vi "SpinCoaterArray2String_v03.vi"(3 "Time Start":dbl[unit], 4 "Program Spin Coater\nSpeed (rpm)          Time (s)":dbl[][](array[numeric])) -> (0 "Prg Spin Coater small":dbl[][](array[numeric]), 1 "remote control String":string)   [LabVIEW 2018, in "SpinCoater.lvclass"]
uses:
  <instrlib>/Classes/SpinCoater/SpinCoater.lvclass
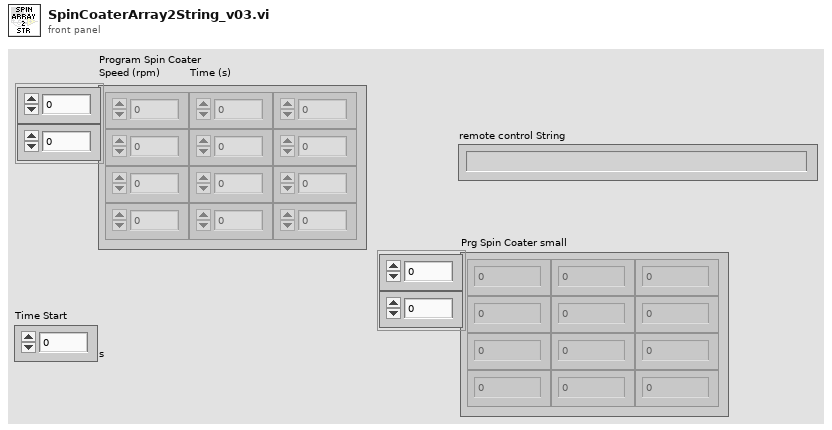
[diagram p1: front panel]
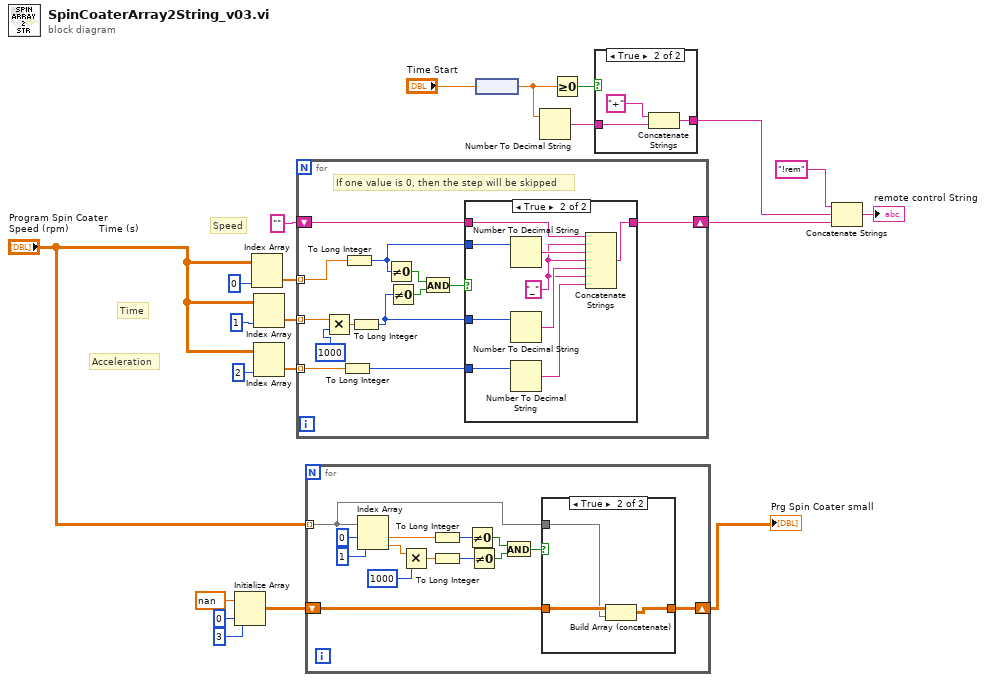
[diagram p0: block diagram]
diagram:
  # "Acceleration"
  # "Time"
  # "Speed"
  n1 = Initialize Array(nan ("element"), 0 ("dimension size"), 3 ("dimension size")) -> (w2:dbl[][])
  n2 = Index Array(array="Program Spin Coater\nSpeed (rpm)          Time (s)", index (col)=0 ("disabled index (col)")) -> (element=w19:dbl[])  [unwired: 1 in]
  n3 = Index Array(array="Program Spin Coater\nSpeed (rpm)          Time (s)", index (col)=1 ("disabled index (col)")) -> (element=w18:dbl[])  [unwired: 1 in]
  n4 = Index Array(array="Program Spin Coater\nSpeed (rpm)          Time (s)", index (col)=2 ("disabled index (col)")) -> (element=w7:dbl[])  [unwired: 1 in]
  n5 = for {
    tunnel: w19 -> [w31] mode=indexing
    tunnel: w18 -> [w24] mode=indexing
    shift-right: [w28] -> w9
    shift-left: "" ("string") -> [w29]
    tunnel: w7 -> [w27] mode=indexing
    # "If one value is 0, then the step will be skipped"
    n6 = Multiply(x=w24, y=1000) -> (x*y=w25:dbl)
    n7 = To Long Integer(number=w27) -> (32bit integer=w26:i32)
    n8 = To Long Integer(number=w31) -> (32bit integer=w30:i32)
    n9 = To Long Integer(number=w25) -> (32bit integer=w22:i32)
    n10 = Not Equal To 0?(x=w30) -> (x != 0?=w34:bool)
    n11 = Not Equal To 0?(x=w22) -> (x != 0?=w33:bool)
    n12 = And(x=w34, y=w33) -> (x .and. y?=w32:bool)
    n13 = case shown="True" w32 {
      tunnel: w30 -> [_ w44]
      tunnel: w22 -> [_ w43]
      tunnel: w29 -> [w35 w40]
      tunnel: [w35 w39] -> w28
      tunnel: w26 -> [_ w38]
      frame False {
      }
      frame True {
        w37 = "_" ("string")
        n14 = Number To Decimal String(number=w44) -> (decimal integer string=w42:string)  [unwired: 1 in]
        n15 = Number To Decimal String(number=w43) -> (decimal integer string=w41:string)  [unwired: 1 in]
        n16 = Number To Decimal String(number=w38) -> (decimal integer string=w36:string)  [unwired: 1 in]
        n17 = Concatenate Strings(w40, w37, w42, w37, w41, w37, w36) -> (w39:string)
      }
    }
  }
  n18 = for {
    tunnel: "Program Spin Coater\nSpeed (rpm)          Time (s)" -> [w50] mode=indexing
    shift-right: [w48] -> w1
    shift-left: w2 -> [w49]
    n19 = Index Array(array=w50, index #1=0 ("index"), index #2=1 ("index")) -> (element #1=w56:dbl, element #2=w46:dbl)
    n20 = Multiply(x=w46, y=1000) -> (x*y=w47:dbl)
    n21 = To Long Integer(number=w56) -> (32bit integer=w52:i32)
    n22 = To Long Integer(number=w47) -> (32bit integer=w53:i32)
    n23 = Not Equal To 0?(x=w52) -> (x != 0?=w55:bool)
    n24 = Not Equal To 0?(x=w53) -> (x != 0?=w54:bool)
    n25 = And(x=w55, y=w54) -> (x .and. y?=w51:bool)
    n26 = case shown="True" w51 {
      tunnel: w50 -> [_ w61]
      tunnel: w49 -> [w59 w62]
      tunnel: [w59 w60] -> w48
      frame False {
      }
      frame True {
        n27 = Build Array (concatenate)(w62, w61) -> (w60:dbl[][])
      }
    }
  }
  "Prg Spin Coater small" <- w1
  n28 = node("Time Start") -> (w13:dbl)
  n29 = Number To Decimal String(number=w13) -> (decimal integer string=w12:string)  [unwired: 1 in]
  n30 = Greater Or Equal To 0?(x=w13) -> (x >= 0?=w14:bool)
  n31 = case shown="True" w14 {
    tunnel: w12 -> [w63 w65]
    tunnel: [w63 w64] -> w11
    frame False {
    }
    frame True {
      n32 = Concatenate Strings("+", w65) -> (w64:string)
    }
  }
  n33 = Concatenate Strings("!rem" ("string"), w11, w9) -> (→"remote control String":string)
